vi "Query ACLR.vi"(8 "error in (no error)":errorcluster, 11 "SA-FSW in":refnum<class "SA-FSW.lvclass">) -> (0 "error out":errorcluster, 1 "ACLR":dbl[](array[numeric]), 2 "Channel Power [dBm]":dbl[](array[numeric]), 3 "SA-FSW out":refnum<class "SA-FSW.lvclass">)   [LabVIEW 2020, in "SA-FSW.lvclass"]
uses:
  SA-FSW.lvclass
  C:/Sandbox/RF Bench/Source Code/WiSpry Test Framework/Instruments/Instrument.lvclass
  Instrument.lvclass/Instrument.ctl
  Instrument.lvclass
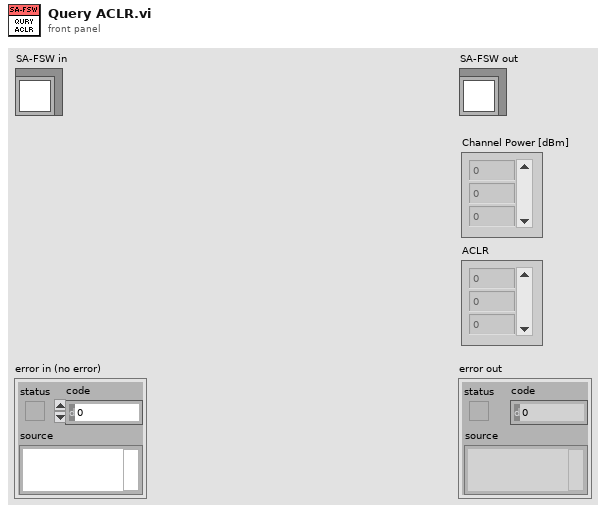
[diagram p1: front panel]
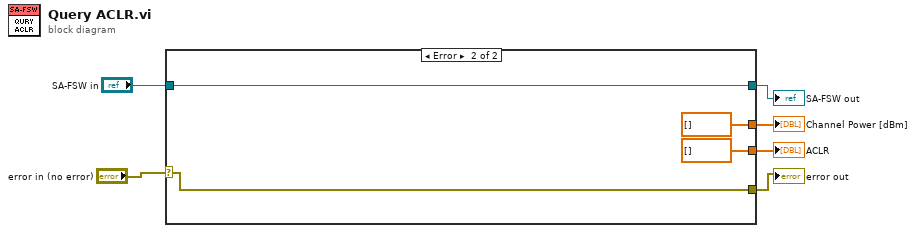
[diagram p0: block diagram]
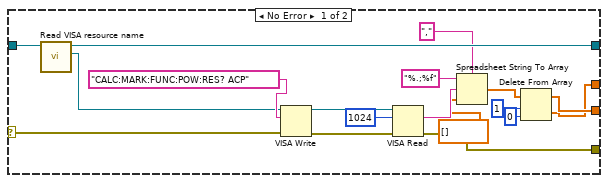
[diagram p2: hidden frame]
diagram:
  n1 = case shown="Error" "error in (no error)" {
    selector: "error in (no error)" -> [w20 w26]
    tunnel: "SA-FSW in" -> [w24 w25]
    tunnel: [w23 w25] -> w1
    tunnel: [w9 dbl[] []] -> w4
    tunnel: [w8 dbl[] []] -> w3
    tunnel: [w7 w26] -> w2
    frame No Error {
      n2 = call "Read VISA resource name.vi"("Instrument in"=w24) -> ("VISA resource name"=w21:refnum<visa-resource-name>, "Instrument out"=w23:refnum<class "SA-FSW.lvclass">)  [unwired: 9 in]
      n3 = VISA Write(VISA resource name=w21, write buffer="CALC:MARK:FUNC:POW:RES? ACP", error in (no error)=w20) -> (VISA resource name out=w18:refnum<visa-resource-name>, error out=w19:errorcluster)  [unwired: 1 out]
      n4 = VISA Read(VISA resource name=w18, byte count=u32 1024, error in (no error)=w19) -> (read buffer=w14:string, error out=w7:errorcluster)  [unwired: 2 out]
      n5 = Spreadsheet String To Array(delimiter (Tab)=",", format string="%.;%f", spreadsheet string=w14, array type (2D Dbl)=dbl[] []) -> (array=w13:dbl[])
      n6 = Delete From Array(array=w13, length=1, index=0) -> (deleted portion=w8:dbl[], array with subset deleted=w9:dbl[])
    }
    frame Error {
    }
  }
  "error out" <- w2
  "SA-FSW out" <- w1
  "ACLR" <- w4
  "Channel Power [dBm]" <- w3
